vi "NISE.remote.Write Register (Core).vi"(0 "SLSC Remote in":refnum<class "SLSC Interface.lvclass">, 1 "type":enum16{"U8", "U16", "U32", "U64"}(ring), 5 "device":refnum<k21>="$DefaultDevices", 7 "register address":u32 format="%.0x", 9 "data":u64 format="%.0x", 11 "error in (no error)":errorcluster) -> (4 "SLSC Remote out":refnum<class "SLSC Interface.lvclass">, 6 "device out":refnum<k21>, 8 "next register address":u32 format="%.0x", 15 "error out":errorcluster)   [LabVIEW 2016, in "SLSC Interface.lvclass"]
uses:
  SLSC Interface Class/SLSC Interface.lvclass
  SLSC Interface Class/SLSC Interface.lvclass/SLSC Interface.ctl
  SLSC Interface Class/NISE.Read client handle.vi
  SLSC Interface Class/NISE.Read URL.vi
  <vilib>/NI/JSON Support for LabVIEW/JSON Data Classes/JSON Object/JSON Object.lvclass
  C:/Program Files (x86)/National Instruments/LabVIEW 2016/vi.lib/NI/JSON Support for LabVIEW/JSON Data Classes/JSON Datatype/JSON Null.lvclass
  SLSC Interface Class/NISE.Read session.vi
  <vilib>/NI/JSON Support for LabVIEW/JSON Data Classes/JSON Object/New JSON Object (Empty).vi
  <vilib>/NI/JSON Support for LabVIEW/JSON Data Classes/JSON Object/Insert Key Value Pair (Single String).vi
  <vilib>/NI/JSON Support for LabVIEW/JSON Data Classes/JSON Object/Insert Key Value Pair (Single Numeric).vi
  <vilib>/NI/NI JSONRPC Server Framework/Classes/Server/Format Client Request (Auto-Increment).vi
  <vilib>/httpClient/POSTBuffer.vi
  <vilib>/NI/NI JSONRPC Server Framework/Classes/Server/Parse Response (Object).vi
  <vilib>/NI/JSON Support for LabVIEW/JSON Data Classes/JSON Object/Get Value (Numeric Value).vi
  <vilib>/NI/NI JSONRPC Server Framework/Classes/Server/JSONRPC Server.lvclass
  <vilib>/httpClient/LabVIEWHTTPClient.lvlib
  <vilib>/NI/JSON Support for LabVIEW/JSON Data Classes/JSON Helper/JSON Helper.lvclass
  C:/Program Files (x86)/National Instruments/LabVIEW 2016/vi.lib/NI/JSON Support for LabVIEW/JSON Data Classes/JSON Structured Type/JSON Structure.lvclass
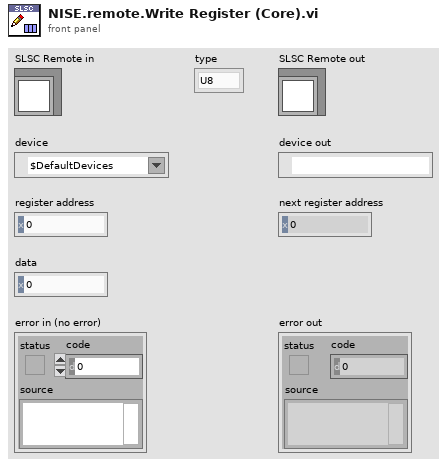
[diagram p1: front panel]
types:
  T1 = typedef "LabVIEWHTTPClient.lvlib/ClientHandle.ctl" = refnum<k1>
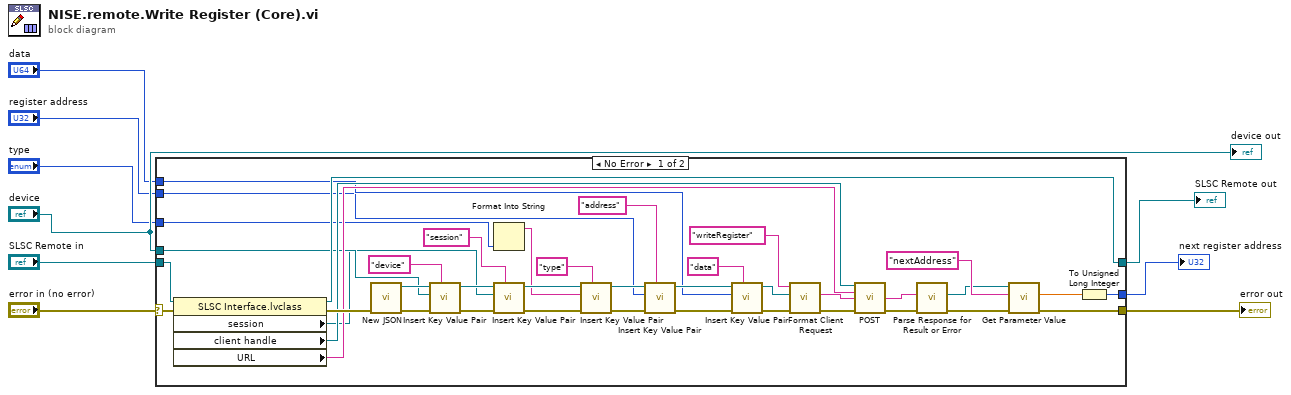
[diagram p0: block diagram]
diagram:
  n1 = case shown="No Error" "error in (no error)" {
    selector: "error in (no error)" -> [w47 w50]
    tunnel: "device" -> [w15 _]
    tunnel: "SLSC Remote in" -> [w49 w51]
    tunnel: [w48 w51] -> w8
    tunnel: [w26 w50] -> w2
    tunnel: "type" -> [w31 _]
    tunnel: "register address" -> [w13 _]
    tunnel: "data" -> [w14 _]
    tunnel: [w25 _] -> w3
    frame No Error {
      n2 = property class="SLSC Interface.lvclass"(reference=w49, error in=w47) -> (reference out=w48:refnum<class "SLSC Interface.lvclass">, error out=w46:errorcluster, "session"=w11:refnum<k21>, "client handle"=w41:T1, "URL"=w40:string)
      n3 = call-poly <vilib>:"New JSON.vi"("error in (no error)"=w46) -> ("error out"=w45:errorcluster, "JSON Object out"=w20:refnum<class "JSON Object.lvclass">)  [unwired: 9 in]
      n4 = call-poly <vilib>:"Insert Key Value Pair.vi"("key"="device" ("Name"), "error in (no error)"=w45, "value"=w15, "JSON Object in"=w20) -> ("error out"=w44:errorcluster, "JSON Object out"=w19:refnum<class "JSON Object.lvclass">)  [unwired: 5 in, 1 out]
      n5 = Format Into String(w31) -> (resulting string=w12:string)  [unwired: 3 in, 1 out]
      n6 = call-poly <vilib>:"Insert Key Value Pair.vi"("key"="session" ("Name"), "error in (no error)"=w44, "value"=w11, "JSON Object in"=w19) -> ("error out"=w32:errorcluster, "JSON Object out"=w18:refnum<class "JSON Object.lvclass">)  [unwired: 5 in, 1 out]
      n7 = call-poly <vilib>:"Insert Key Value Pair.vi"("key"="type" ("Name"), "error in (no error)"=w32, "value"=w12, "JSON Object in"=w18) -> ("error out"=w36:errorcluster, "JSON Object out"=w17:refnum<class "JSON Object.lvclass">)  [unwired: 5 in, 1 out]
      n8 = call-poly <vilib>:"Insert Key Value Pair.vi"("key"="address" ("Name"), "error in (no error)"=w36, "value"=w13, "JSON Object in"=w17) -> ("error out"=w33:errorcluster, "JSON Object out"=w16:refnum<class "JSON Object.lvclass">)  [unwired: 5 in, 1 out]
      n9 = call-poly <vilib>:"Insert Key Value Pair.vi"("key"="data" ("Name"), "error in (no error)"=w33, "value"=w14, "JSON Object in"=w16) -> ("error out"=w35:errorcluster, "JSON Object out"=w34:refnum<class "JSON Object.lvclass">)  [unwired: 5 in, 1 out]
      n10 = call-poly <vilib>:"Format Client Request.vi"("error in (no error)"=w35, "JSON in"=w34, "method"="writeRegister") -> ("error out"=w39:errorcluster, "Request String"=w42:string)  [unwired: 7 in]
      n11 = call-poly <vilib>:"POST.vi"("client handle"=w41, "url"=w40, "buffer"=w42, "error in (no error)"=w39) -> ("body"=w38:string, "error out"=w37:errorcluster)  [unwired: 8 in, 2 out]
      n12 = call-poly <vilib>:"Parse Response for Result or Error.vi"("error in"=w37, "Response String In"=w38) -> ("error out"=w28:errorcluster, "JSON Array"=w10:refnum<class "JSON Object.lvclass">)  [unwired: 7 in, 1 out]
      n13 = call-poly <vilib>:"Get Parameter Value.vi"("error in (no error)"=w28, "key"="nextAddress" ("Parameter Name"), "JSON Object in"=w10) -> ("error out"=w26:errorcluster, "value"=w24:dbl)  [unwired: 7 in]
      n14 = To Unsigned Long Integer(number=w24) -> (unsigned 32bit integer=w25:u32)
    }
    frame Error {
    }
  }
  "error out" <- w2
  "SLSC Remote out" <- w8
  "next register address" <- w3
  "device out" <- "device"
